vi "DSF Configuration Cluster to File.vi"(8 "error in (no error)":errorcluster, 10 "framework configuration":T1, 11 "dsf configuration file path":path) -> (0 "error out":errorcluster, 3 "dsf configuration file path dup":path)   [LabVIEW 2017, in "DSF Core.lvlib" / "Configuration Session.lvclass"]
uses:
  Configuration Session.lvclass
  Typedefs/DSF Engine Framework Configuration.ctl
  Typedefs/DSF Engine Plugin Configuration.ctl
  Typedefs/DSF Timing Info.ctl
  Typedefs/DSF Engine Plugin Thread Configuration.ctl
  Typedefs/DSF Settings Info.ctl
  Typedefs/DSF Engine Transfer Group Configuration.ctl
  Typedefs/DSF Direction.ctl
  Typedefs/DSF Engine Transfer Configuration.ctl
  Typedefs/DSF Byte Order.ctl
  Typedefs/DSF Engine Channel Configuration.ctl
  Typedefs/DSF Data Type.ctl
  Typedefs/DSF Timeout Behavior.ctl
  Typedefs/DSF Plugin Info.ctl
  Typedefs/DSF Group Info.ctl
  Typedefs/DSF Transfer Info.ctl
  Typedefs/DSF Channel Info.ctl
  Write Channel.vi
  Write Transfer.vi
  Write Group.vi
  Write Plugin.vi
  DSF Core.lvlib
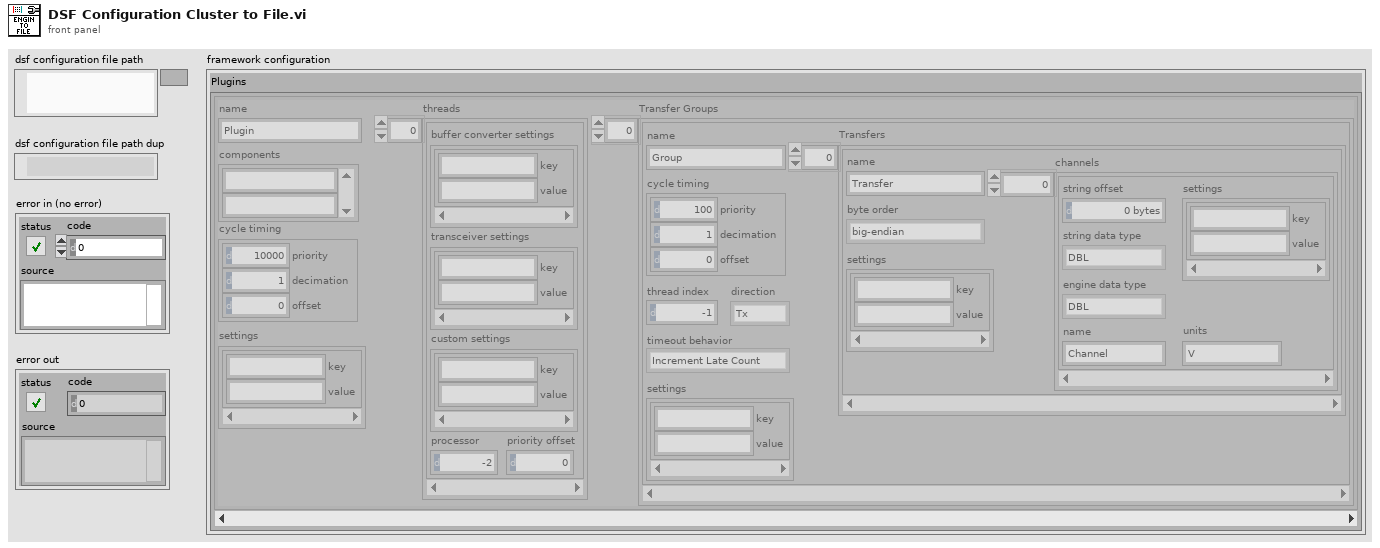
[diagram p1: front panel]
types:
  T1 = typedef "DSF Core.lvlib/DSF Engine Framework Configuration.ctl" = cluster{"Plugins":T2[]}
  T2 = typedef "DSF Core.lvlib/DSF Engine Plugin Configuration.ctl" = cluster{"name":string, "components":string[], "cycle timing":T3, "threads":T4[], "Transfer Groups":T6[], "settings":T5}
  T3 = typedef "DSF Core.lvlib/DSF Timing Info.ctl" = cluster{"priority":u64, "decimation":u64, "offset":u64}
  T4 = typedef "DSF Core.lvlib/DSF Engine Plugin Thread Configuration.ctl" = cluster{"buffer converter settings":T5, "transceiver settings":T5, "custom settings":T5, "processor":i32, "priority offset":i16}
  T5 = typedef "DSF Core.lvlib/DSF Settings Info.ctl" = cluster{"key":string, "value":string}[]
  T6 = typedef "DSF Core.lvlib/DSF Engine Transfer Group Configuration.ctl" = cluster{"name":string, "direction":T7, "cycle timing":T3, "thread index":i32, "settings":T5, "Transfers":T8[], "timeout behavior":T12}
  T7 = typedef "DSF Core.lvlib/DSF Direction.ctl" = enum8{"Tx", "Rx"}
  T8 = typedef "DSF Core.lvlib/DSF Engine Transfer Configuration.ctl" = cluster{"name":string, "byte order":T9, "settings":T5, "channels":T10[]}
  T9 = typedef "DSF Core.lvlib/DSF Byte Order.ctl" = enum8{"big-endian", "little-endian"}
  T10 = typedef "DSF Core.lvlib/DSF Engine Channel Configuration.ctl" = cluster{"string offset":u64, "string data type":T11, "engine data type":T11, "name":string, "settings":T5, "units":string}
  T11 = typedef "DSF Core.lvlib/DSF Data Type.ctl" = enum8{"Bool", "SGL", "DBL", "I8", "I16", "I32", "I64", "U8", "U16", "U32", "U64"}
  T12 = typedef "DSF Core.lvlib/DSF Timeout Behavior.ctl" = enum8{"Increment Late Count", "Throw Error"}
  T13 = typedef "DSF Core.lvlib/DSF Plugin Info.ctl" = cluster{"components":string[], "timing":T3, "group ids":string[], "settings id":string, "threads":T4[]}
  T14 = typedef "DSF Core.lvlib/DSF Group Info.ctl" = cluster{"direction":T7, "timing":T3, "transfer ids":string[], "settings id":string, "thread":i32, "timeout behavior":T12}
  T15 = typedef "DSF Core.lvlib/DSF Transfer Info.ctl" = cluster{"byte order":T9, "channel ids":string[], "settings id":string}
  T16 = typedef "DSF Core.lvlib/DSF Channel Info.ctl" = cluster{"string buffer offset":u64, "string data type":T11, "engine data type":T11, "settings id":string, "units":string}
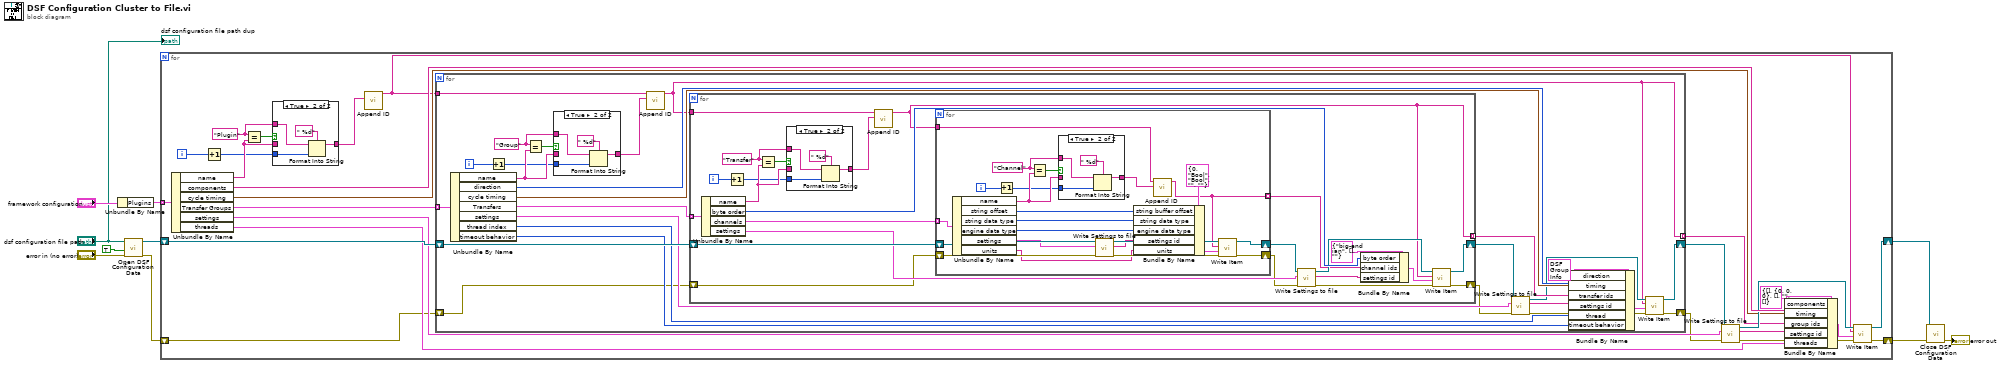
[diagram p0: block diagram]
diagram:
  n1 = Unbundle By Name("framework configuration") -> ("Plugins"=w7:T2[])
  n2 = call "Open DSF Configuration Data.vi"("error in (no error)"="error in (no error)", "replace if found? (F)"=TRUE, "dsf configuration file path"="dsf configuration file path") -> ("error out"=w1:errorcluster, "Configuration Session"=w6:refnum<class "Configuration Session.lvclass">)  [unwired: 4 in, 3 out]
  n3 = for {
    tunnel: w7 -> [w35] mode=indexing
    shift-right: [w29] -> w5
    shift-left: w6 -> [w30]
    shift-right: [w21] -> w2
    shift-left: w1 -> [w17]
    i -> [w12]
    w15 = "Plugin" ("x")
    n4 = Unbundle By Name(w35) -> ("name"=w14:string, "components"=w32:string[], "cycle timing"=w19:T3, "Transfer Groups"=w31:T6[], "settings"=w27:T5, "threads"=w20:T4[])
    n5 = Increment(x=w12) -> (x+1=w11:i32)
    n6 = Equal?(x=w15, y=w14) -> (x = y?=w16:bool)
    n7 = case shown="True" w16 {
      tunnel: [w36 w40] -> w13
      tunnel: w14 -> [w36 _]
      tunnel: w15 -> [_ w39]
      tunnel: w11 -> [_ w37]
      frame False {
      }
      frame True {
        n8 = Format Into String(format string=" %d", initial string=w39, w37) -> (resulting string=w40:string)  [unwired: 1 in, 1 out]
      }
    }
    n9 = call "Append ID.vi"("name"=w13) -> ("appended id string"=w18:string)  [unwired: 10 in]
    n10 = for {
      tunnel: w31 -> [w67] mode=indexing
      shift-right: [w59] -> w25
      shift-left: w30 -> [w61]
      tunnel: [w48] -> w24 mode=indexing
      tunnel: w18 -> [w49]
      shift-right: [w55] -> w23
      shift-left: w17 -> [w47]
      i -> [w42]
      w45 = "Group" ("x")
      n11 = Unbundle By Name(w67) -> ("name"=w44:string, "direction"=w64:T7, "cycle timing"=w63:T3, "Transfers"=w62:T8[], "settings"=w58:T5, "thread index"=w52:i32, "timeout behavior"=w50:T12)
      n12 = Increment(x=w42) -> (x+1=w41:i32)
      n13 = Equal?(x=w45, y=w44) -> (x = y?=w46:bool)
      n14 = case shown="True" w46 {
        tunnel: [w68 w72] -> w43
        tunnel: w44 -> [w68 _]
        tunnel: w45 -> [_ w71]
        tunnel: w41 -> [_ w69]
        frame False {
        }
        frame True {
          n15 = Format Into String(format string=" %d", initial string=w71, w69) -> (resulting string=w72:string)  [unwired: 1 in, 1 out]
        }
      }
      n16 = call "Append ID.vi"("name"=w43, "initial id string (\"\")"=w49) -> ("appended id string"=w48:string)  [unwired: 9 in]
      n17 = for {
        tunnel: w62 -> [w96] mode=indexing
        shift-right: [w89] -> w60
        shift-left: w61 -> [w91]
        tunnel: [w79] -> w56 mode=indexing
        tunnel: w48 -> [w80]
        shift-right: [w81] -> w54
        shift-left: w47 -> [w84]
        i -> [w74]
        w77 = "Transfer" ("x")
        n18 = Unbundle By Name(w96) -> ("name"=w76:string, "byte order"=w94:T9, "channels"=w92:T10[], "settings"=w87:T5)
        n19 = Increment(x=w74) -> (x+1=w73:i32)
        n20 = Equal?(x=w77, y=w76) -> (x = y?=w78:bool)
        n21 = case shown="True" w78 {
          tunnel: [w97 w101] -> w75
          tunnel: w76 -> [w97 _]
          tunnel: w77 -> [_ w100]
          tunnel: w73 -> [_ w98]
          frame False {
          }
          frame True {
            n22 = Format Into String(format string=" %d", initial string=w100, w98) -> (resulting string=w101:string)  [unwired: 1 in, 1 out]
          }
        }
        n23 = call "Append ID.vi"("name"=w75, "initial id string (\"\")"=w80) -> ("appended id string"=w79:string)  [unwired: 9 in]
        n24 = for {
          tunnel: w92 -> [w124] mode=indexing
          shift-right: [w121] -> w90
          shift-left: w91 -> [w119]
          tunnel: [w110] -> w85 mode=indexing
          tunnel: w79 -> [w105]
          shift-right: [w120] -> w83
          shift-left: w84 -> [w118]
          i -> [w103]
          w106 = "Channel" ("x")
          n25 = Unbundle By Name(w124) -> ("name"=w104:string, "string offset"=w111:u64, "string data type"=w112:T11, "engine data type"=w113:T11, "settings"=w117:T5, "units"=w109:string)
          n26 = Increment(x=w103) -> (x+1=w102:i32)
          n27 = Equal?(x=w106, y=w104) -> (x = y?=w108:bool)
          n28 = case shown="True" w108 {
            tunnel: [w125 w129] -> w107
            tunnel: w104 -> [w125 _]
            tunnel: w106 -> [_ w128]
            tunnel: w102 -> [_ w127]
            frame False {
            }
            frame True {
              n29 = Format Into String(format string=" %d", initial string=w128, w127) -> (resulting string=w129:string)  [unwired: 1 in, 1 out]
            }
          }
          n30 = call "Write Settings to file.vi"("error in (no error)"=w118, "settings"=w117, "Configuration Session in"=w119) -> ("error out"=w115:errorcluster, "settings id"=w114:string, "Configuration Session out"=w116:refnum<class "Configuration Session.lvclass">)  [unwired: 6 in]
          n31 = Bundle By Name(cluster=T16 {"string buffer offset"=0, "string data type"=enum."Bool", "engine data type"=enum."Bool", "settings id"="", "units"=""} ("values"), "string buffer offset"=w111, "string data type"=w112, "engine data type"=w113, "settings id"=w114, "units"=w109) -> (w122:T16)
          n32 = call "Append ID.vi"("name"=w107, "initial id string (\"\")"=w105) -> ("appended id string"=w110:string)  [unwired: 9 in]
          n33 = call-poly "Write Item.vi"("error in (no error)"=w115, "channel values"=w122, "id"=w110, "Configuration Session in"=w116) -> ("error out"=w120:errorcluster, "Configuration Session out"=w121:refnum<class "Configuration Session.lvclass">)  [unwired: 5 in, 1 out]
        }
        n34 = call "Write Settings to file.vi"("error in (no error)"=w83, "settings"=w87, "Configuration Session in"=w90) -> ("error out"=w82:errorcluster, "settings id"=w86:string, "Configuration Session out"=w88:refnum<class "Configuration Session.lvclass">)  [unwired: 6 in]
        n35 = Bundle By Name(cluster=T15 {"byte order"=enum."big-endian", "channel ids"=[], "settings id"=""} ("values"), "byte order"=w94, "channel ids"=w85, "settings id"=w86) -> (w93:T15)
        n36 = call-poly "Write Item.vi"("error in (no error)"=w82, "transfer values"=w93, "id"=w79, "Configuration Session in"=w88) -> ("error out"=w81:errorcluster, "Configuration Session out"=w89:refnum<class "Configuration Session.lvclass">)  [unwired: 5 in, 1 out]
      }
      n37 = call "Write Settings to file.vi"("error in (no error)"=w54, "settings"=w58, "Configuration Session in"=w60) -> ("error out"=w53:errorcluster, "settings id"=w57:string, "Configuration Session out"=w51:refnum<class "Configuration Session.lvclass">)  [unwired: 6 in]
      n38 = Bundle By Name(cluster=T14 {"direction"=enum."Tx", "timing"={"priority"=0, "decimation"=0, "offset"=0}, "transfer ids"=[], "settings id"="", "thread"=0, "timeout behavior"=enum."Increment Late Count"} ("group values"), "direction"=w64, "timing"=w63, "transfer ids"=w56, "settings id"=w57, "thread"=w52, "timeout behavior"=w50) -> (w65:T14)
      n39 = call-poly "Write Item.vi"("error in (no error)"=w53, "group values"=w65, "id"=w48, "Configuration Session in"=w51) -> ("error out"=w55:errorcluster, "Configuration Session out"=w59:refnum<class "Configuration Session.lvclass">)  [unwired: 5 in, 1 out]
    }
    n40 = call "Write Settings to file.vi"("error in (no error)"=w23, "settings"=w27, "Configuration Session in"=w25) -> ("error out"=w22:errorcluster, "settings id"=w28:string, "Configuration Session out"=w26:refnum<class "Configuration Session.lvclass">)  [unwired: 6 in]
    n41 = Bundle By Name(cluster=T13 {"components"=[], "timing"={"priority"=0, "decimation"=0, "offset"=0}, "group ids"=[], "settings id"="", "threads"=[]} ("plugin values"), "components"=w32, "timing"=w19, "group ids"=w24, "settings id"=w28, "threads"=w20) -> (w33:T13)
    n42 = call-poly "Write Item.vi"("error in (no error)"=w22, "plugin values"=w33, "id"=w18, "Configuration Session in"=w26) -> ("error out"=w21:errorcluster, "Configuration Session out"=w29:refnum<class "Configuration Session.lvclass">)  [unwired: 5 in, 1 out]
  }
  n43 = call "Close DSF Configuration Data.vi"("error in (no error)"=w2, "Configuration Session"=w5) -> ("error out"=→"error out":errorcluster)  [unwired: 8 in, 1 out]
  "dsf configuration file path dup" <- "dsf configuration file path"
